vi "Value Change Test.vi"() -> ()   [LabVIEW 2016]
uses:
  XControls/Reference/VI Reference.xctl
panel:
  in  "VI Reference":refnum<vi>(xcontrol)
  in  "stop":bool
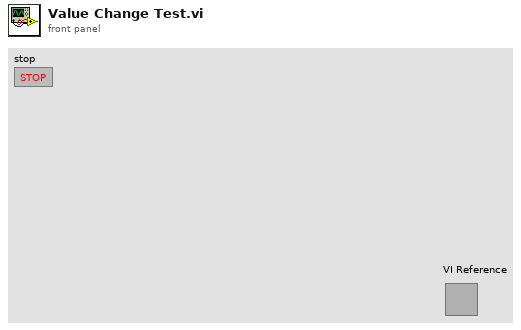
[diagram p1: front panel]
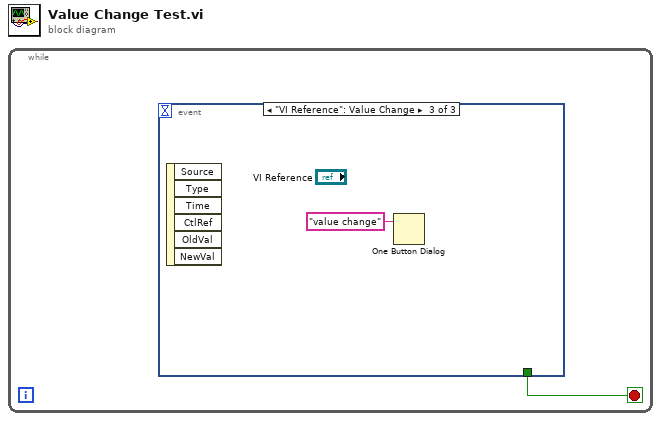
[diagram p0: block diagram]
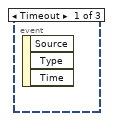
[diagram p2: hidden frame]
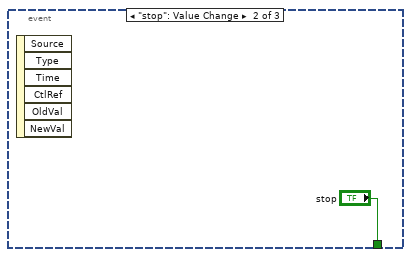
[diagram p3: hidden frame]
diagram:
  n1 = while {
    stop <- w1 stop-if-true
    n2 = event shown="[2] \"VI Reference\": Value Change" {
      selector: _ -> [_ _ _]
      dyn-events: _ -> [_ _ _]
      timeout: _ -> [_ _ _]
      tunnel: [_ "stop" _] -> w1
      event Timeout {
        n3 = event-data() -> ()  [unwired: 1 in, 3 out]
      }
      event "stop": Value Change {
        n4 = event-data() -> ()  [unwired: 1 in, 6 out]
      }
      event "VI Reference": Value Change {
        n5 = event-data() -> ()  [unwired: 1 in, 6 out]
        n6 = One Button Dialog(message="value change") -> ()  [unwired: 1 in, 1 out]
      }
    }
  }
